vi "create Food.vi"(8 "error in (no error)":errorcluster, 9 "Point Value":u32, 10 "Starting Point":cluster{"x":u32, "y":u32}, 11 "Food in":refnum<class "Food.lvclass">) -> (0 "error out":errorcluster, 3 "Food out":refnum<class "Food.lvclass">)   [LabVIEW 2020, in "Food.lvclass"]
uses:
  Food.lvclass
  Food.lvclass/Food.ctl
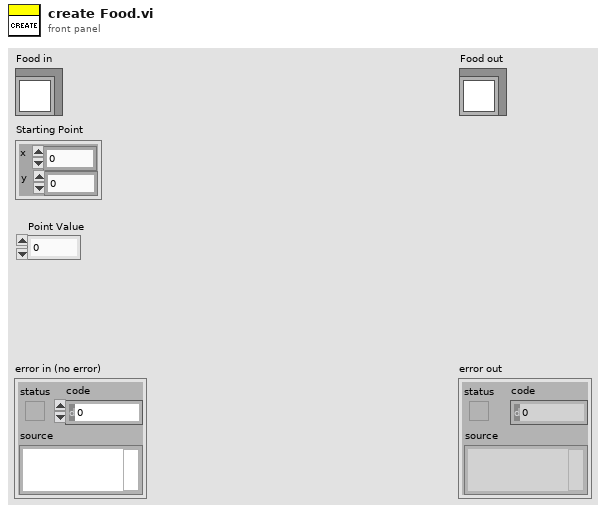
[diagram p1: front panel]
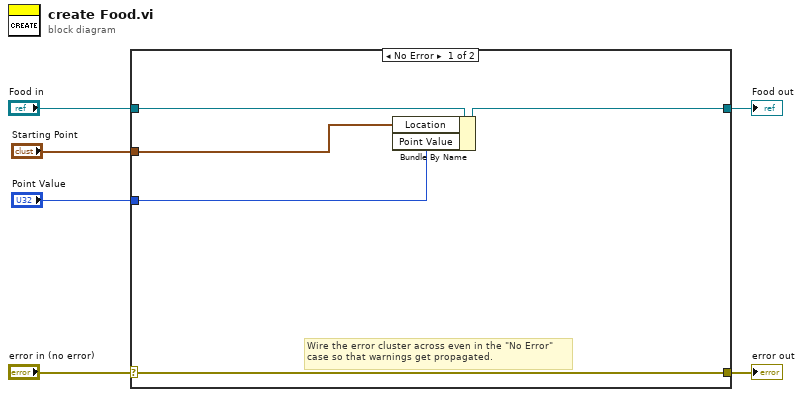
[diagram p0: block diagram]
diagram:
  n1 = case shown="No Error" "error in (no error)" {
    selector: "error in (no error)" -> [w10 w13]
    tunnel: [w10 w13] -> w5
    tunnel: [w9 w12] -> w3
    tunnel: "Food in" -> [w11 w12]
    tunnel: "Point Value" -> [w8 _]
    tunnel: "Starting Point" -> [w7 _]
    frame No Error {
      # "Wire the error cluster across even in the \"No Error\"\ncase so that warnings get propagated."
      n2 = Bundle By Name(cluster=w11, "Location"=w7, "Point Value"=w8) -> (w9:refnum<class "Food.lvclass">)
    }
    frame Error {
    }
  }
  "error out" <- w5
  "Food out" <- w3
